vi "Merge Data.vi"(8 "error in (no error)":errorcluster, 10 "From":refnum<class "Server Message.lvclass">, 11 "Server Message in":refnum<class "Server Message.lvclass">) -> (0 "error out":errorcluster, 3 "Server Message out":refnum<class "Server Message.lvclass">)   [LabVIEW 2020, in "obs-websocket.lvlib" / "Server Message.lvclass"]
uses:
  Server Message.lvclass
  Server Message.lvclass/Server Message.ctl
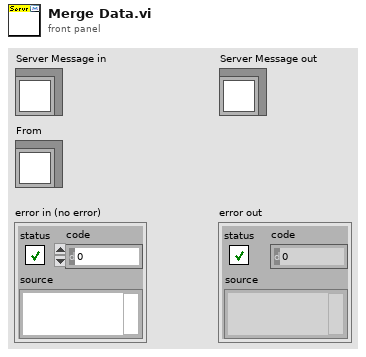
[diagram p1: front panel]
types:
  T1 = typedef "obs-websocket.lvlib/Server Operation.ctl" = enum16{"Hello", "Identified", "Event", "RequestResponse", "RequestBatchResponse"}
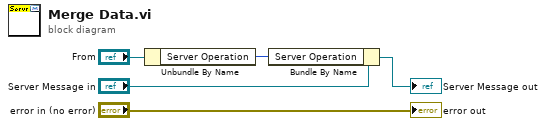
[diagram p0: block diagram]
diagram:
  n1 = Unbundle By Name("From") -> ("Server Operation"=w1:T1)
  n2 = Bundle By Name(cluster="Server Message in", "Server Operation"=w1) -> (→"Server Message out":refnum<class "Server Message.lvclass">)
  "error out" <- "error in (no error)"
